vi "GlobalVariables.vi"() -> ()   [LabVIEW 2011]
uses:
  Motors/MotorStateType.ctl
  Motors/MotorPosType.ctl
  Typedefs/XYf.ctl
  Typedefs/MeasureConfigType.ctl
  Typedefs/MeasureConfigOutputMode.ctl
  qtrk/QTrkLVBinding/QTrkSettings.ctl
  Typedefs/TrackingConfigType.ctl
  qtrk/QTrkLVBinding/QTrkLocalizationType.ctl
  qtrk/QTrkLVBinding/QTrkZCommandType.ctl
  ExperimentProgram/ExperimentProgramType.ctl
  ExperimentProgram/ExProgCommandType.ctl
  ExperimentProgram/ExProgCommandEnumType.ctl
  Motors/MotorAxisEnum.ctl
  Motors/MotorPosFlagsType.ctl
  Camera/GenericCameraConfigType.ctl
  Typedefs/QueueListType.ctl
  Typedefs/Cmd_MotorIn.ctl
  Typedefs/CmdEnum_MotorIn.ctl
  Typedefs/CmdData_NewFrame.ctl
  <vilib>/vision/Image Controls.llb/IMAQ Image.ctl
  Typedefs/CmdEnum_CameraFrameType.ctl
  Typedefs/UserInterfaceEventType.ctl
  Typedefs/CmdEnum_UserInterfaceCmd.ctl
  ExperimentProgram/ScriptEventType.ctl
  Motors/MotorConfigType.ctl
  Camera/CameraInstance.ctl
  Modules/CameraInterface/CameraInterface.ctl
  Modules/CameraInterface/CICloseType.ctl
  Modules/CameraInterface/CIGetSetGenericConfig.ctl
  Modules/CameraInterface/CIGrabType.ctl
  Modules/CameraInterface/CISettingsDlg.ctl
  Modules/CameraInterface/CIAdjustBeadPos.ctl
  Modules/CameraInterface/CISaveLoadSettings.ctl
  Camera/PixelCalibrationDataType.ctl
panel:
  in  "Timing settings":T1={"Script loop delay"=100, "Motor loop "=50, "Motor get pos wait time\nper axis"=2}
  in  "Pixel calibration":T2
  in  "Main view framerate":i32=30
  in  "Main View Grab loop running?":bool
  out "Main Camera Instance":T4
  in  "Update motor positions?":bool
  out "MotorConfig":T12={"Offset"={"Magnet Z"=0.0, "Magnet rotation"=0.0, "Camera"={"X"=0.0, "Y"=0.0}, "Piezo XY"={"X"=0.0, "Y"=0.0}, "Piezo Z"=0.0}, "Maximum pos"={"Magnet Z"=0.0, "Magnet rotation"=0.0, "Camera"={"X"=0.0, "Y"=0.0}, "Piezo XY"={"X"=0.0, "Y"=0.0}, "Piezo Z"=0.0}, "Min limited?"={"Magnet Z"=FALSE, "Magnet rotation"=FALSE, "Camera"={"X"=FALSE, "Y"=FALSE}, "Piezo XY"={"X"=FALSE, "Y"=FALSE}, "Piezo Z"=FALSE}, "Max limited?"={"Magnet Z"=FALSE, "Magnet rotation"=FALSE, "Camera"={"X"=FALSE, "Y"=FALSE}, "Piezo XY"={"X"=FALSE, "Y"=FALSE}, "Piezo Z"=FALSE}, "Has velocity support"={"Magnet Z"=TRUE, "Magnet rotation"=TRUE, "Camera"={"X"=FALSE, "Y"=FALSE}, "Piezo XY"={"X"=FALSE, "Y"=FALSE}, "Piezo Z"=FALSE}, "Default velocity"={"Magnet Z"=0.0, "Magnet rotation"=0.0, "Camera"={"X"=0.0, "Y"=0.0}, "Piezo XY"={"X"=0.0, "Y"=0.0}, "Piezo Z"=0.0}}
  out "Queue List":T16
  out "MeasureConfig":T17={"Bead locations"=[{"X"=0, "Y"=0}], "ROI"=200, "Experiment base path"=path "", "Image output subdir"="images", "Output mode"=enum."None", "Traces output subdir"="traces", "QTrk Settings"={"Image width"=150, "Image height"=150, "Number of threads (CPU based)"=-1, "CUDA Device"=-2, "COM Background correction factor"=0.0, "ZLUT MinRadius"=8.0, "ZLUT Radial sample density"=5.0, "ZLUT Angular sample density"=2.0, "ZLUT ROI Coverage"=0.7, "QI Iterations"=1, "QI MinRadius"=2.0, "QI Radial sample density"=5.0, "QI Angular sample density"=2.0, "QI ROI Coverage"=0.7, "QI Angular Step \nIteration Factor"=0.8, "XCOR Profile Length"=1, "XCOR Profile Width"=128, "XCOR Iterations"=32, "Gaussian 2D Fit Iterations"=2, "Gaussian 2D Sigma (pixels)"=3.0, "Downsample"=0}, "Tracking Config"={"Number of steps"=0, "ZLUT stepsize (um)"=0.0, "Z correction factor"=0.0, "Start piezo Z (um)"=0.0, "Pixel size (nm)"=0.0, "2D Localization Type"=enum."Quadrant Interpolation", "Z Command (None)"=enum."Nothing", "Z Piezo scale"=FALSE, "ZLUT Building\nimages per frame"=0, "ZLUT Bias correction planes"=1}, "Experiment Name"="", "Program"={"Commands"=[], "Motor Axis accuracy conditions"={"Magnet Z"=0.0, "Magnet rotation"=0.0, "Camera"={"X"=0.0, "Y"=0.0}, "Piezo XY"={"X"=0.0, "Y"=0.0}, "Piezo Z"=0.0}, "Axis flags"={"Magnet Z"=FALSE, "Magnet rotation"=FALSE, "Camera"={"X"=FALSE, "Y"=FALSE}, "Piezo XY"={"X"=FALSE, "Y"=FALSE}, "Piezo Z"=FALSE}}, "ZLUT"=[], "Camera settings"={"Framerate (Hz)"=60, "Exposure time (us)"=5000, "Image size"={"Width"=1280, "Height"=1024}, "Number of buffers"=30}, "Experiment Script"="", "Max frames in memory"=10000, "Save traces as binary"=FALSE, "Pixel Calibration Gain Image"="camera_calib_gain.bin", "Pixel Calibration Offset Image"="camera_calib_offset.bin", "Use pixel calibration images"=FALSE, "Internal camera settings"="", "Trace write interval"=100} {"QTrk Settings"."QI ROI Coverage" format="%_2g"; "QTrk Settings"."QI MinRadius" format="%.2f"; "QTrk Settings"."QI Angular sample density" format="%.3f"; "QTrk Settings"."QI Radial sample density" format="%.2f"; "QTrk Settings"."ZLUT Radial sample density" format="%.2f"; "QTrk Settings"."ZLUT MinRadius" format="%.2f"}
  in  "MotorState":T28
  in  "Quit app":bool
  # "(used for commands with string parameters)"
  # "-2: Use all devices\n-1: Use best device"
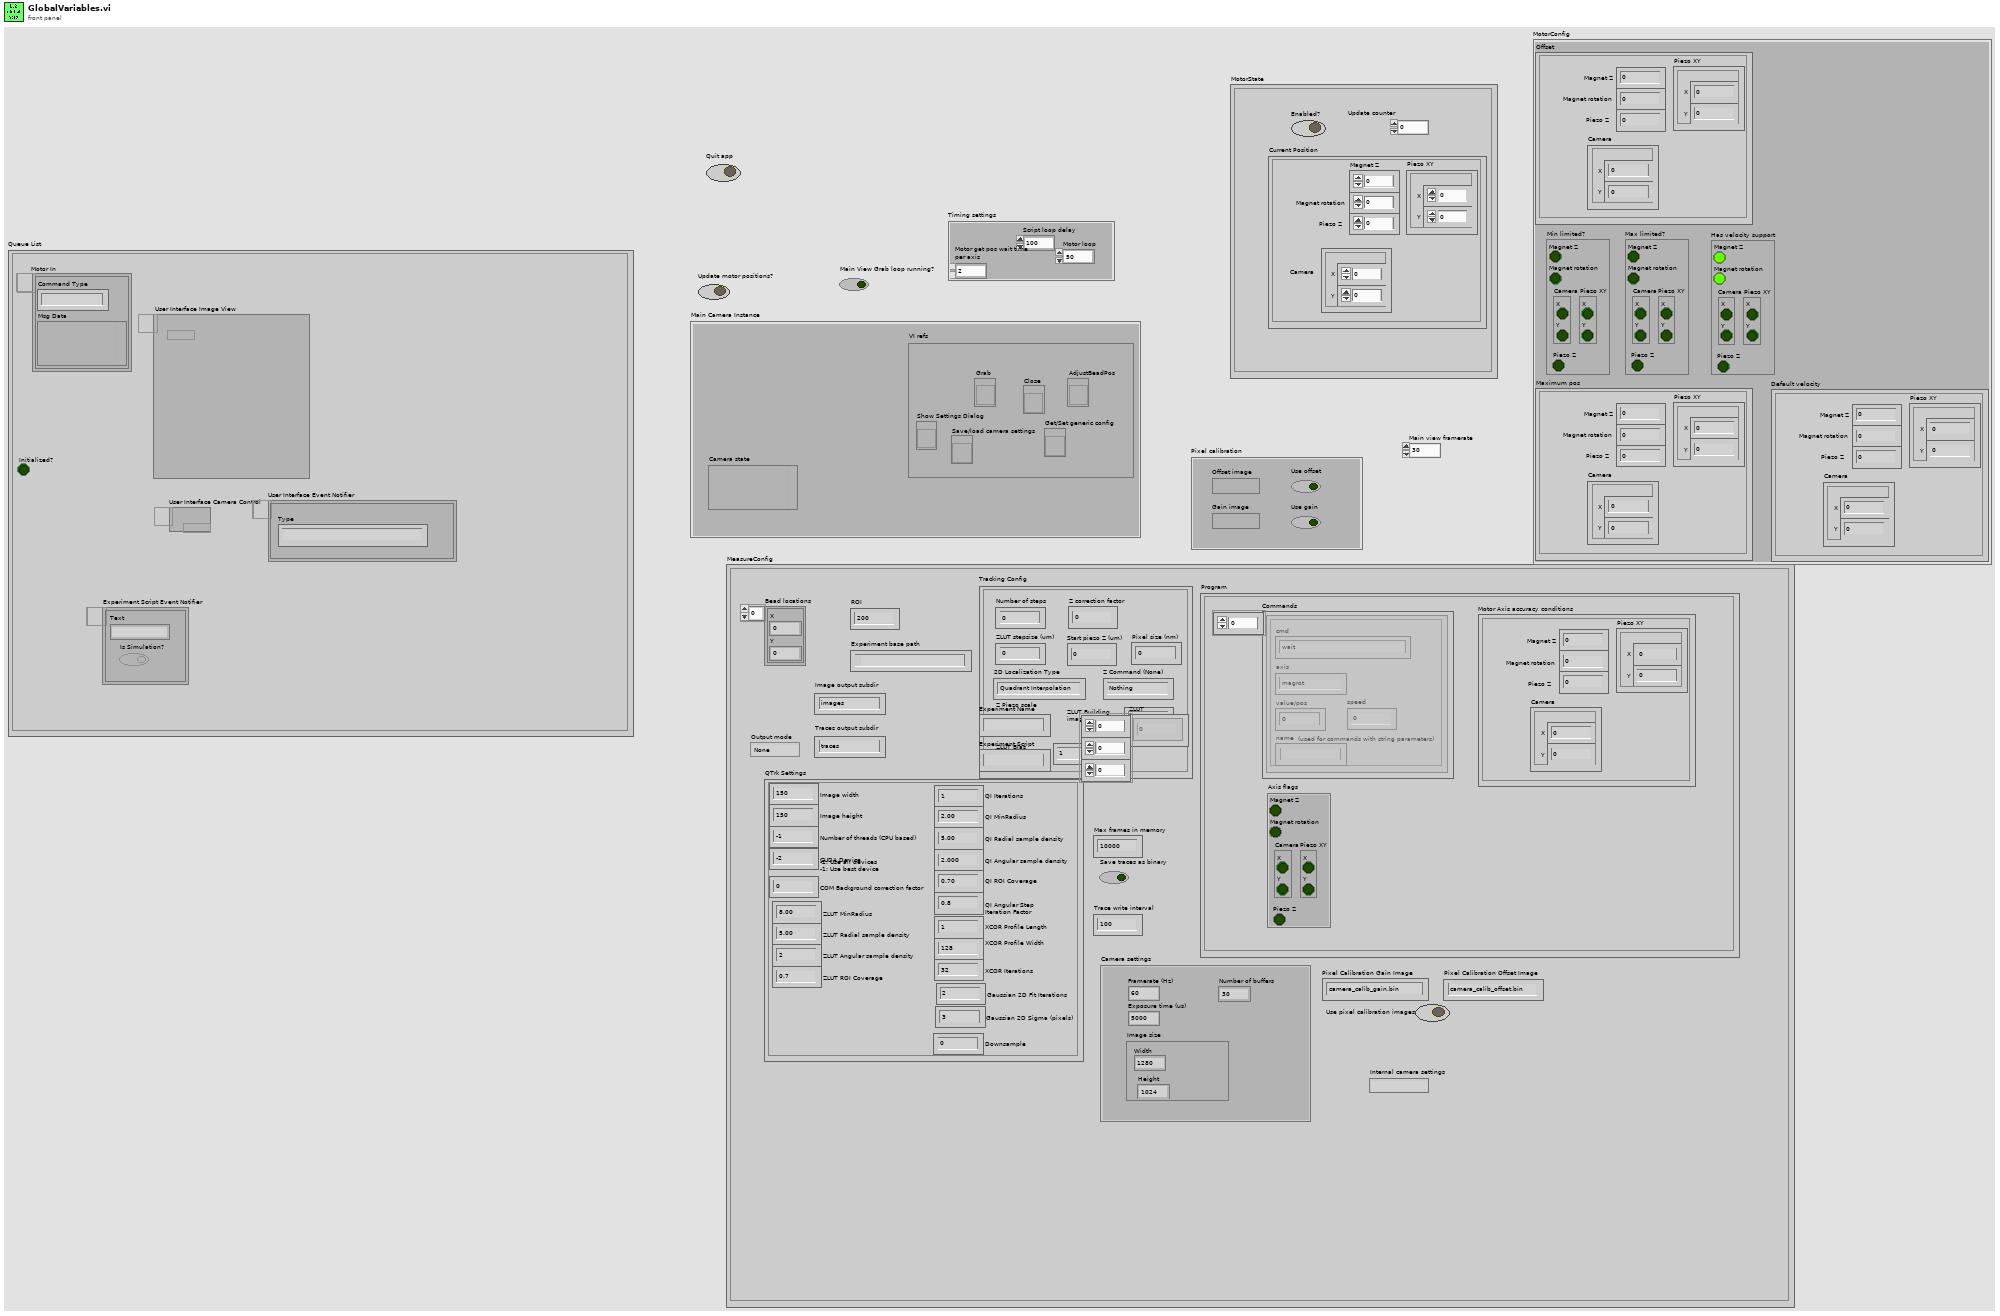
[diagram p1: front panel]
types:
  T1 = cluster{"Script loop delay":i32, "Motor loop ":i32, "Motor get pos wait time\nper axis":i32}
  T2 = typedef "PixelCalibrationDataType.ctl" = cluster{"Offset image":T3, "Gain image":T3, "Use offset":bool, "Use gain":bool}
  T3 = typedef "IMAQ Image.ctl" = refnum<image>
  T4 = typedef "CameraInstance.ctl" = cluster{"VI refs":T5, "Camera state":variant}
  T5 = typedef "CameraInterface.ctl" = cluster{"Close":T6, "Get/Set generic config":T7, "Grab":T8, "Show Settings Dialog":T9, "AdjustBeadPos":T10, "Save/load camera settings":T11}
  T6 = typedef "CICloseType.ctl" = refnum<vi>
  T7 = typedef "CIGetSetGenericConfig.ctl" = refnum<vi>
  T8 = typedef "CIGrabType.ctl" = refnum<vi>
  T9 = typedef "CISettingsDlg.ctl" = refnum<vi>
  T10 = typedef "CIAdjustBeadPos.ctl" = refnum<vi>
  T11 = typedef "CISaveLoadSettings.ctl" = refnum<vi>
  T12 = typedef "MotorConfigType.ctl" = cluster{"Offset":T13, "Maximum pos":T13, "Min limited?":T15, "Max limited?":T15, "Has velocity support":T15, "Default velocity":T13}
  T13 = typedef "MotorPosType.ctl" = cluster{"Magnet Z":dbl, "Magnet rotation":dbl, "Camera":T14, "Piezo XY":T14, "Piezo Z":dbl}
  T14 = typedef "XYf.ctl" = cluster{"X":sgl, "Y":sgl}
  T15 = typedef "MotorPosFlagsType.ctl" = cluster{"Magnet Z":bool, "Magnet rotation":bool, "Camera":cluster{"X":bool, "Y":bool}, "Piezo XY":cluster{"X":bool, "Y":bool}, "Piezo Z":bool}
  T16 = typedef "QueueListType.ctl" = cluster{"Motor In":refnum<queue>, "User Interface Image View":refnum<queue>, "User Interface Camera Control":refnum<queue>, "User Interface Event Notifier":refnum<notifier>, "Initialized?":bool, "Experiment Script Event Notifier":refnum<notifier>}
  T17 = typedef "MeasureConfigType.ctl" = cluster{"Bead locations":cluster{"X":i32, "Y":i32}[], "ROI":i32, "Experiment base path":path, "Image output subdir":string, "Output mode":T18, "Traces output subdir":string, "QTrk Settings":T19, "Tracking Config":T20, "Experiment Name":string, "Program":T23, "ZLUT":sgl[][][], "Camera settings":T27, "Experiment Script":string, "Max frames in memory":i32, "Save traces as binary":bool, "Pixel Calibration Gain Image":string, "Pixel Calibration Offset Image":string, "Use pixel calibration images":bool, "Internal camera settings":string, "Trace write interval":i32}
  T18 = typedef "MeasureConfigOutputMode.ctl" = enum16{"None", "Track", "SaveImages"}
  T19 = typedef "QTrkSettings.ctl" = cluster{"Image width":i32, "Image height":i32, "Number of threads (CPU based)":i32, "CUDA Device":i32, "COM Background correction factor":sgl, "ZLUT MinRadius":sgl, "ZLUT Radial sample density":sgl, "ZLUT Angular sample density":sgl, "ZLUT ROI Coverage":sgl, "QI Iterations":i32, "QI MinRadius":sgl, "QI Radial sample density":sgl, "QI Angular sample density":sgl, "QI ROI Coverage":sgl, "QI Angular Step \nIteration Factor":sgl, "XCOR Profile Length":i32, "XCOR Profile Width":i32, "XCOR Iterations":i32, "Gaussian 2D Fit Iterations":i32, "Gaussian 2D Sigma (pixels)":sgl, "Downsample":i32}
  T20 = typedef "TrackingConfigType.ctl" = cluster{"Number of steps":i32, "ZLUT stepsize (um)":sgl, "Z correction factor":sgl, "Start piezo Z (um)":sgl, "Pixel size (nm)":sgl, "2D Localization Type":T21, "Z Command (None)":T22, "Z Piezo scale":bool, "ZLUT Building\nimages per frame":i32, "ZLUT Bias correction planes":i32}
  T21 = typedef "QTrkLocalizationType.ctl" = enum16{"Center-of-Mass", "1D Cross-Correlation", "Quadrant Interpolation", "Gaussian 2D MLE", "QI + ZLUTAlign", "ZLUTAlign", "QI + FourierLUT"}
  T22 = typedef "QTrkZCommandType.ctl" = enum16{"Nothing", "ComputeZ", "BuildRadialZLUT", "BuildImageZLUT", "RadialZLUT+ImageZLUT"}
  T23 = typedef "ExperimentProgramType.ctl" = cluster{"Commands":T24[], "Motor Axis accuracy conditions":T13, "Axis flags":T15}
  T24 = typedef "ExProgCommandType.ctl" = cluster{"cmd":T25, "axis":T26, "value/pos":dbl, "speed":dbl, "name":string}
  T25 = typedef "ExProgCommandEnumType.ctl" = enum16{"wait", "move", "event", "idle", "when", "section", "stop"}
  T26 = typedef "MotorAxisEnum.ctl" = enum16{"no axis", "magrot", "magpos", "px", "py", "pz", "camx", "camy"}
  T27 = typedef "GenericCameraConfigType.ctl" = cluster{"Framerate (Hz)":i32, "Exposure time (us)":i32, "Image size":cluster{"Width":i32, "Height":i32}, "Number of buffers":i32}
  T28 = typedef "MotorStateType.ctl" = cluster{"Enabled?":bool, "Current Position":T13, "Update counter":i32}
diagram:
